vi "Listbox Helper.vi"(10 "Count In":i32, 11 "Display Row":i32) -> (3 "Out":i32)   [LabVIEW 2014]
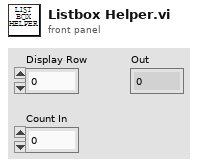
[diagram p1: front panel]
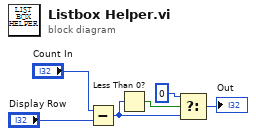
[diagram p0: block diagram]
diagram:
  n1 = Subtract(x="Count In", y="Display Row") -> (x-y=w2:i32)
  n2 = Less Than 0?(x=w2) -> (x < 0?=w1:bool)
  n3 = Select(t=0 ("y"), s=w1, f=w2) -> (s? t:f=→"Out":i32)
